vi "DataTranslation_server.vi"(0 "Board type":T1=enum."DT LV-link", 1 "interval scanning":bool, 2 "Client Time":dbl=3399992102.447224, 5 "No of samples+extra":i32=200 min=0 step=1, 7 "Trigger mode":T2, 9 "output polarity":u16(ring)=1 items=["do not change", "positive", "negative"], 11 "Ch & spans":T3[](array[typedef])=[{"high limit (10V)"=10.0, "low limit (-10V)"=-10.0, "Ch No"=0, "Var name"="RV (Vin)", "Use Latest Calib"=FALSE}] {"low limit (-10V)" format="%.3f"; "high limit (10V)" format="%.3f"}, 12 "Actual Sampling rate (Hz)":dbl=10000.0 format="%.2f", 13 "Local Client?":bool=TRUE, 14 "Current Block No":i32) -> (4 "I16 data":i16[][](array[numeric]), 6 "Block Timings":T4={"Started"=3399991568.753699, "Ended"=3399991587.0837474, "Analogue Frequency Hz"=50000.0} {"Analogue Frequency Hz" format="%.2f"}, 10 "group channel settings":T5(array[cluster])=[{"channel"="", "upper input limits"=0.0, "lower input limits"=0.0, "range"=0.0, "polarity"=0, "gain"=0.0, "coupling"=0, "input mode"=0, "scale multiplier"=1.6666666666666668e-07, "scale offset"=0.0}] {"scale offset" format="%#_16f"; "scale multiplier" format="%#_16f"; "input mode" format="%#_16f"; "coupling" format="%#_16f"; "gain" format="%#_16f"; "polarity" format="%#_16f"; "range" format="%#_16f"; "lower input limits" format="%#_16f"; "upper input limits" format="%#_16f"}, 15 "error out":errorcluster={"status"=TRUE, "code"=1172, "source"="Error calling method LvLink2.LvTask.ReadDblData2DAs1D, (System.Reflection.TargetInvocationException: Exception has been thrown by the target of an invocation.\n\tInner Exception: LvLink2.LvException: Timeout) <append><b>LvLink2.LvException</b> in OLReadMultiple2D.vi->DataTranslation_server.vi->Acquire_Data.vi->Get_data.vi->Measurement.vi"})   [LabVIEW 2010]
uses:
  Controls/Block_start_and_end.ctl
  Data_Translation/DataTranslation_global.vi
  Globals/Meas_global.vi
  <userlib>/LV-Link3/PolySubVIs/DtCreateAinChan.vi
  PWA/PWAtasksGLOBAL.vi
  <userlib>/LV-Link3/PolySubVIs/DtOLTimingSetInput.vi
  <userlib>/LV-Link3/PolySubVIs/DtOLReadMultiple2D.vi
  <userlib>/LV-Link3/PolySubVIs/DtOLTriggerDigital.vi
  Controls/Ch_and_Spans.ctl
  Controls/Trigger_Mode.ctl
  Controls/Board_Types.ctl
panel:
  in  "error in":errorcluster
  out "AFG error out":errorcluster
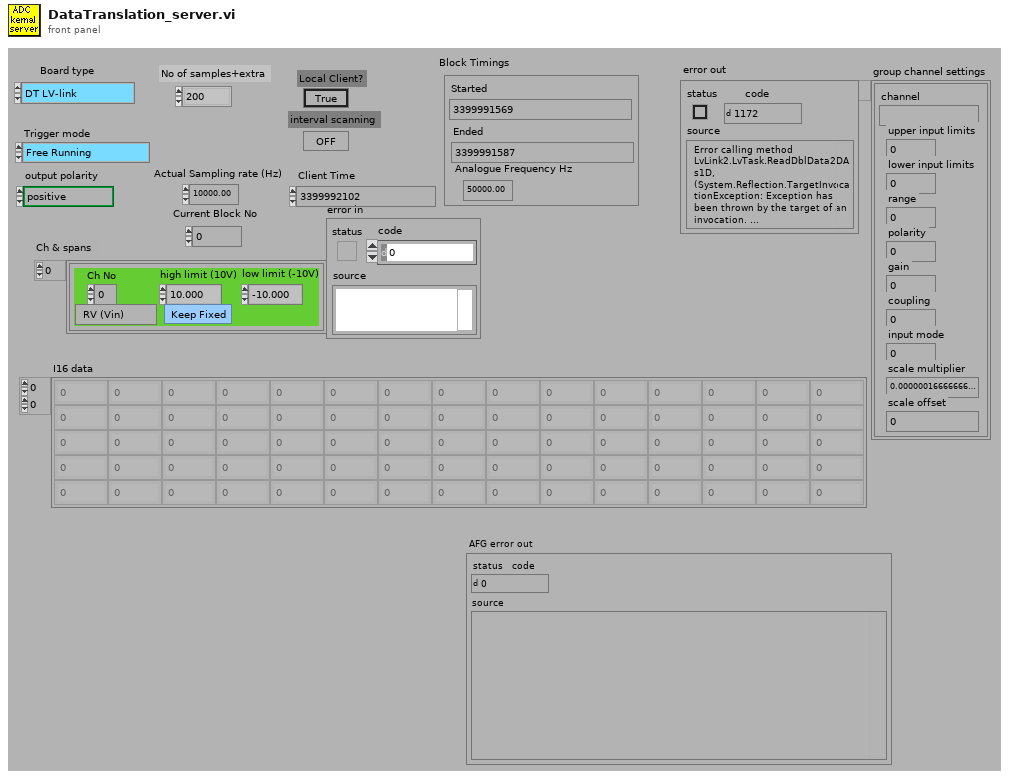
[diagram p1: front panel]
types:
  T1 = typedef "Board_Types.ctl" = enum16{"Simulate", "Local ADAM", "Server ADAM", "NI-DAQmx", "NI-DAQmxBase", "ADC488", "DT LV-link"}
  T2 = typedef "Trigger_Mode.ctl" = enum16{"Free Running", "Start on Trigger", "Trigger Every Block", "Trigger Every Sample"}
  T3 = typedef "Ch_and_Spans.ctl" = cluster{"high limit (10V)":sgl, "low limit (-10V)":sgl, "Ch No":i16, "Var name":string, "Use Latest Calib":bool}
  T4 = typedef "Block_start_and_end.ctl" = cluster{"Started":dbl, "Ended":dbl, "Analogue Frequency Hz":dbl}
  T5 = cluster{"channel":string, "upper input limits":sgl, "lower input limits":sgl, "range":sgl, "polarity":u16, "gain":sgl, "coupling":u16, "input mode":u16, "scale multiplier":dbl, "scale offset":dbl}[]
  T6 = cluster{"channel":string, "upper input limits":sgl, "lower input limits":sgl, "range":sgl, "polarity":u16, "gain":sgl, "coupling":u16, "input mode":u16, "scale multiplier":dbl, "scale offset":dbl}
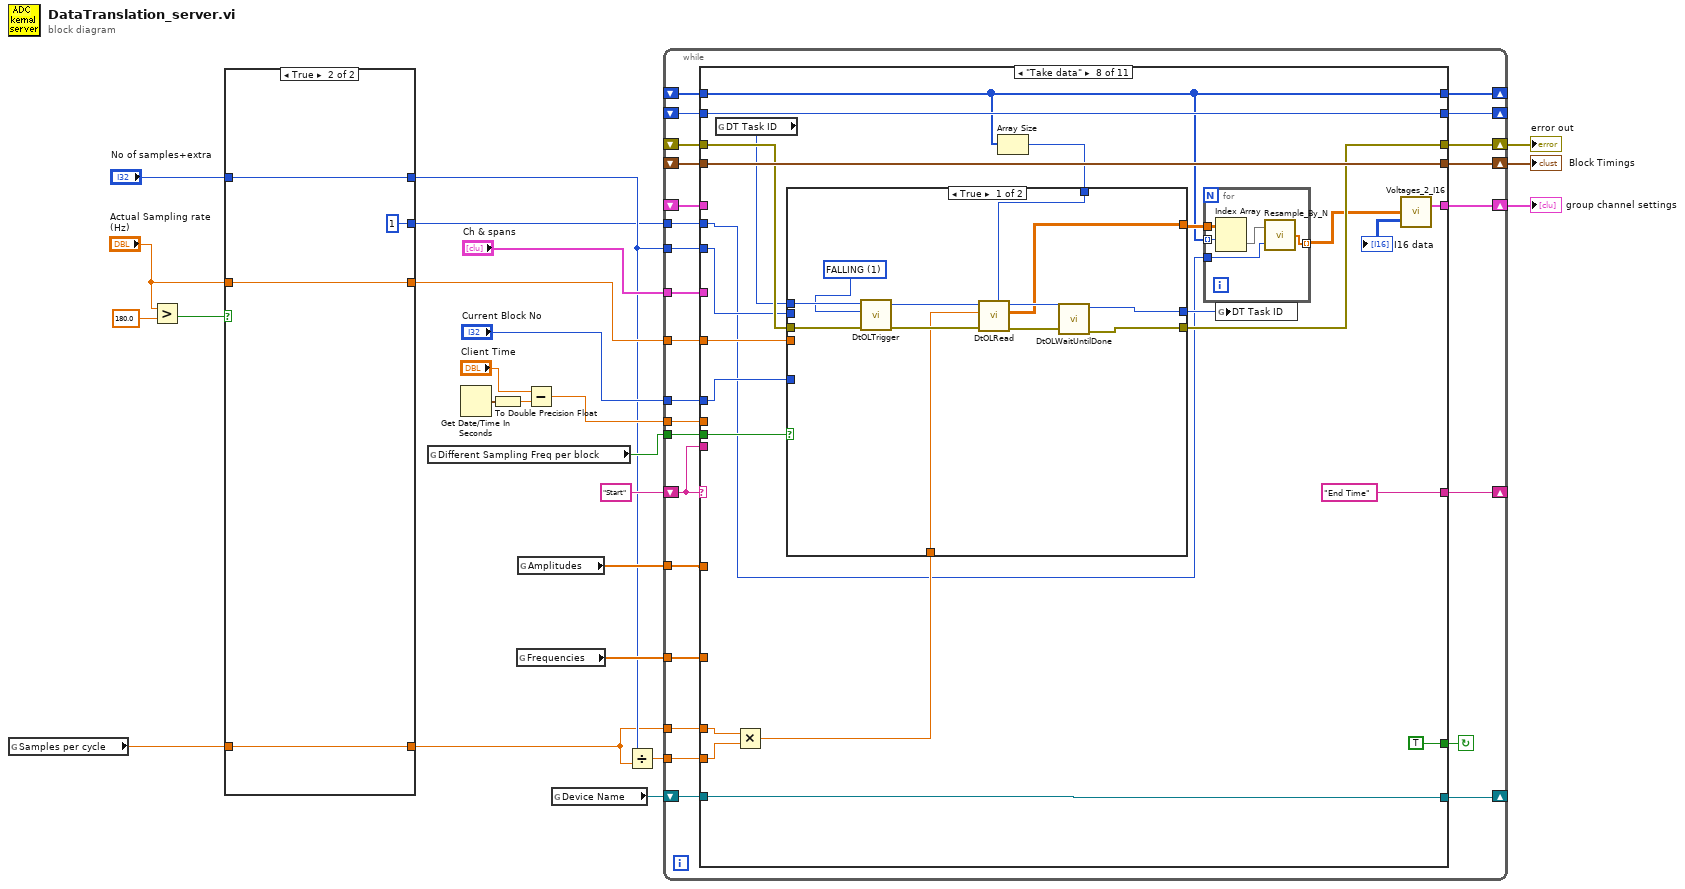
[diagram p0: block diagram]
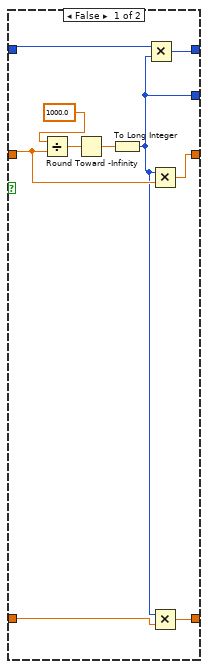
[diagram p2: hidden frame]
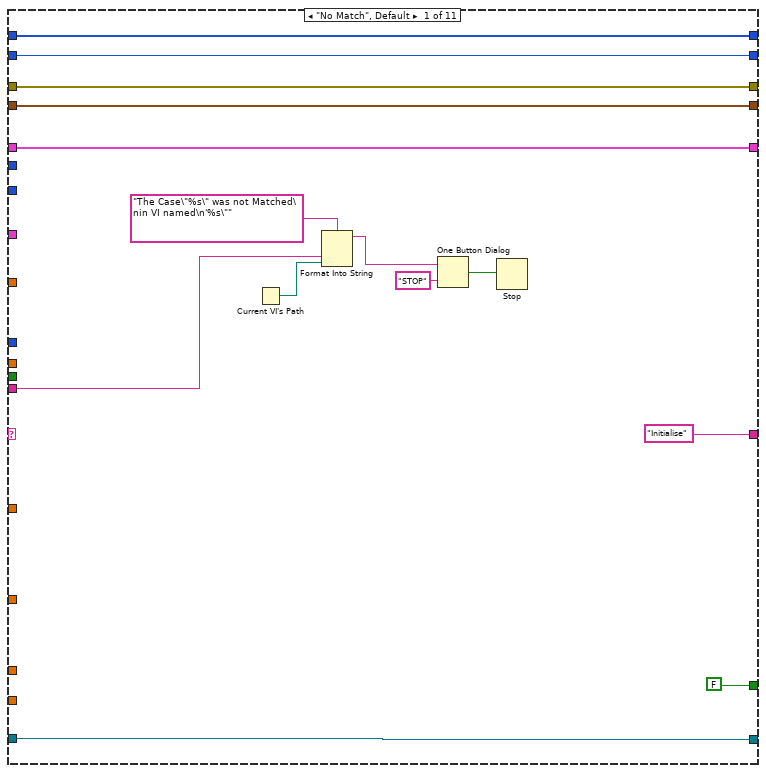
[diagram p3: hidden frame]
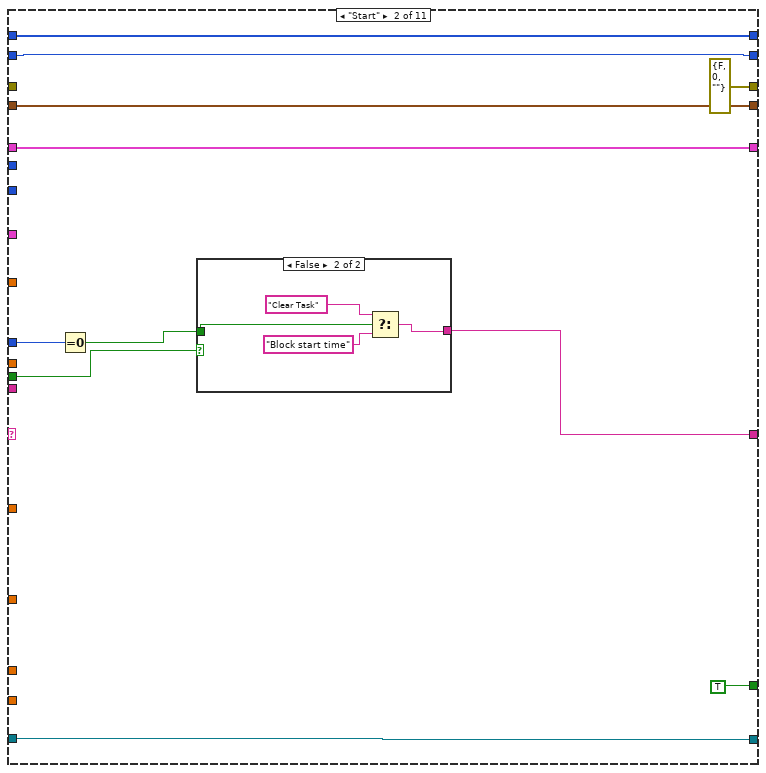
[diagram p4: hidden frame]
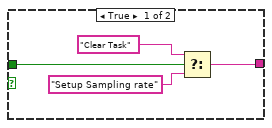
[diagram p5: hidden frame]
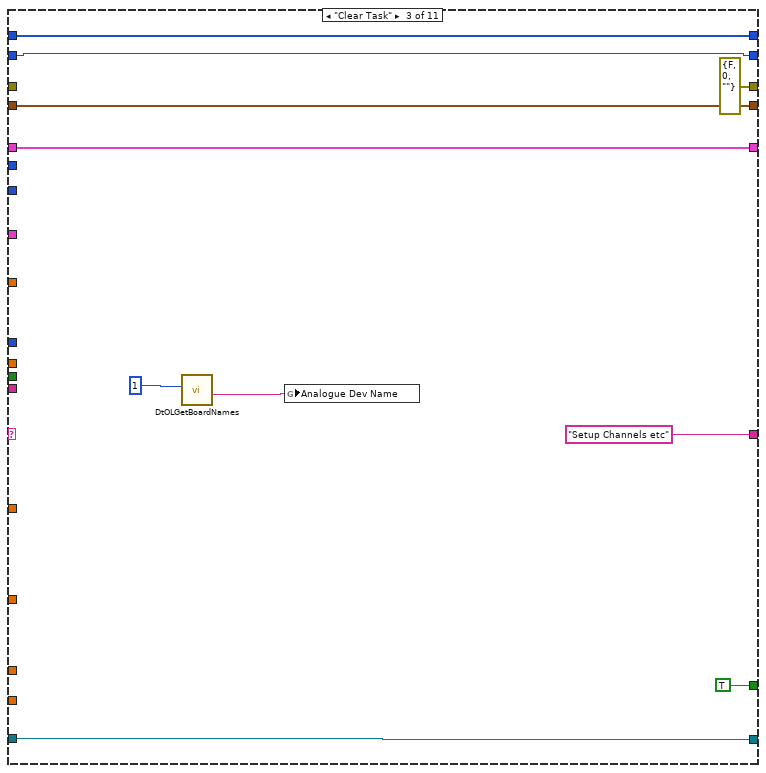
[diagram p6: hidden frame]
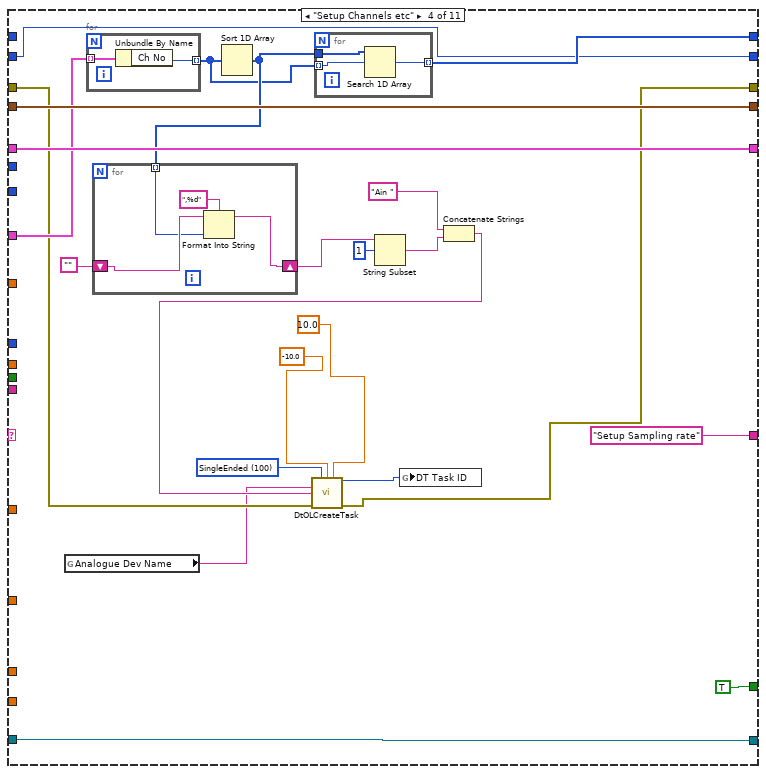
[diagram p7: hidden frame]
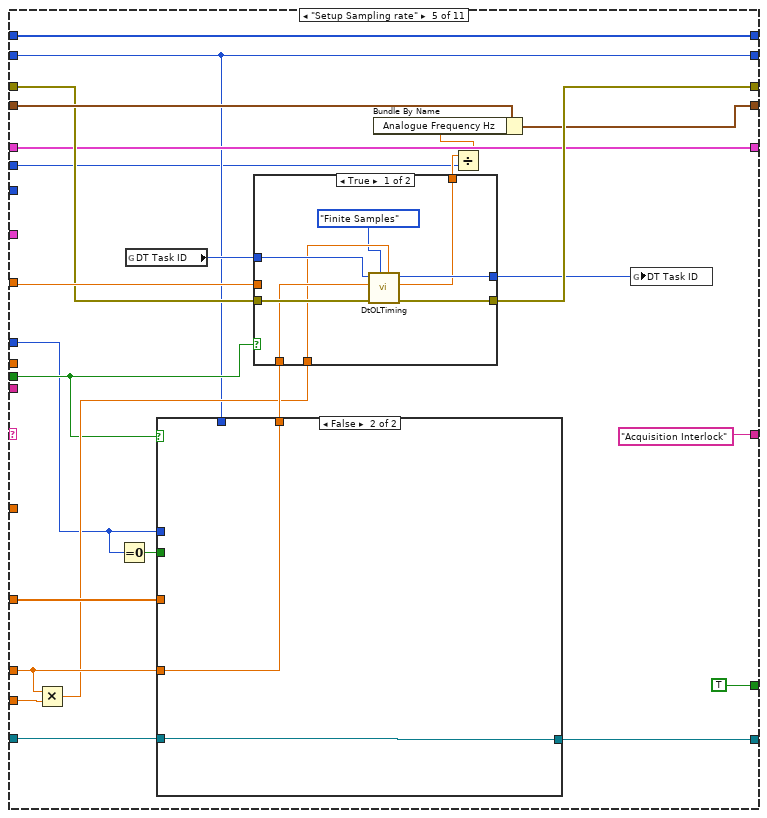
[diagram p8: hidden frame]
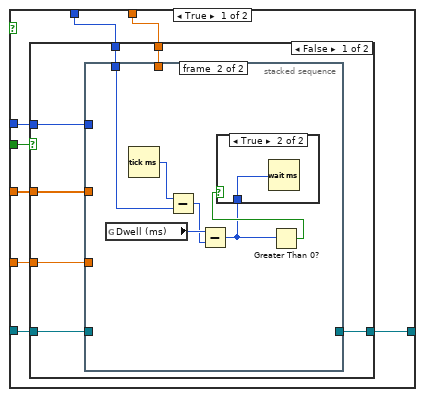
[diagram p9: hidden frame]
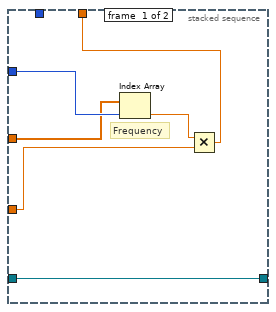
[diagram p10: hidden frame]
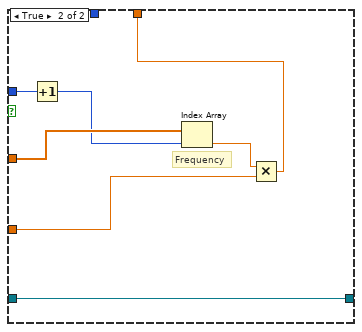
[diagram p12: hidden frame]
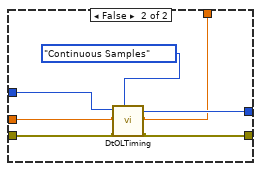
[diagram p13: hidden frame]
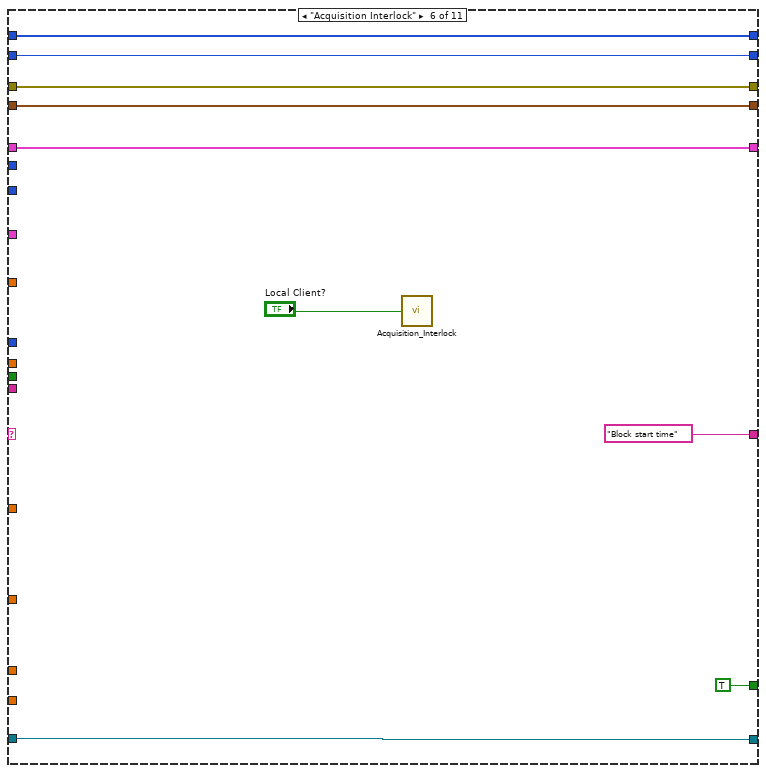
[diagram p14: hidden frame]
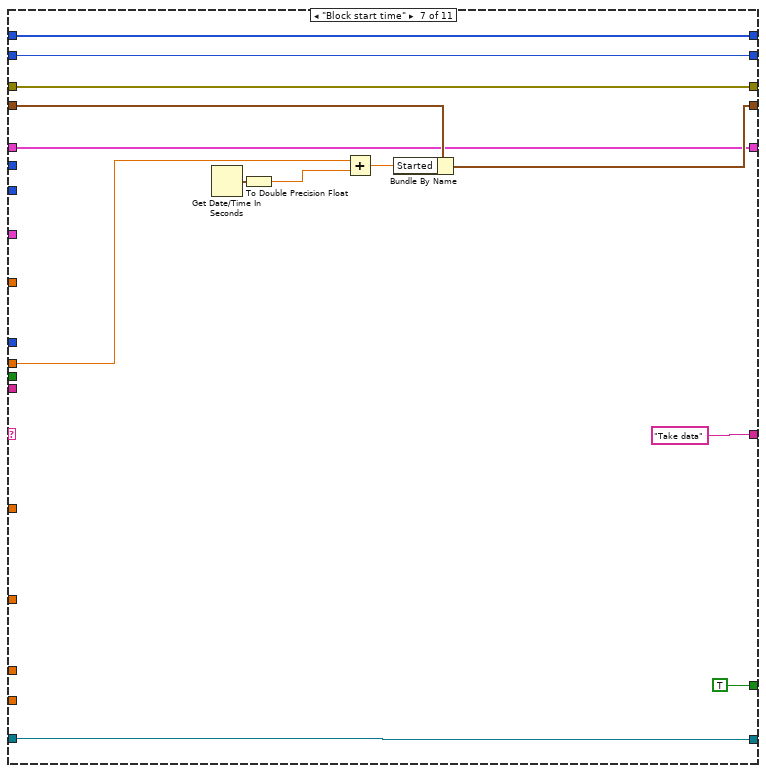
[diagram p15: hidden frame]
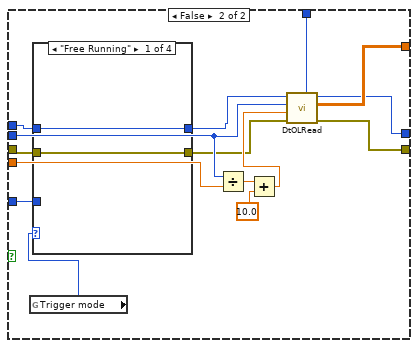
[diagram p16: hidden frame]
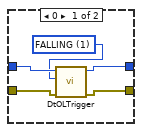
[diagram p18: hidden frame]
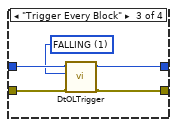
[diagram p19: hidden frame]
diagram:
  n1 = global read "DataTranslation_global.vi" "Samples per cycle"() -> (w2:dbl)
  n2 = Greater?(x="Actual Sampling rate (Hz)", y=180.0) -> (0:w8:bool)
  n3 = case shown="True" w8 {
    tunnel: "Actual Sampling rate (Hz)" -> [w28 w38]
    tunnel: [w29 w38] -> w6
    tunnel: [w31 w37] -> w5
    tunnel: "No of samples+extra" -> [w30 w37]
    tunnel: [w27 w36] -> w3
    tunnel: w2 -> [w26 w36]
    tunnel: [w25 1] -> w1
    frame False {
      n4 = Divide(x=1000.0, y=w28) -> (x/y=w33:dbl)
      n5 = Round Toward -Infinity(1:w33) -> (0:w32:dbl)
      n6 = To Long Integer(number=w32) -> (32bit integer=w25:i32)
      n7 = Multiply(x=w30, y=w25) -> (x*y=w31:i32)
      n8 = Multiply(x=w25, y=w28) -> (x*y=w29:dbl)
      n9 = Multiply(x=w25, y=w26) -> (x*y=w27:dbl)
    }
    frame True {
    }
  }
  n10 = global read "DataTranslation_global.vi" "Different Sampling Freq per block"() -> (w10:bool)
  n11 = Get Date/Time In Seconds() -> (seconds since 1Jan1904=w23:timestamp)
  n12 = To Double Precision Float(number=w23) -> (double precision float=w22:dbl)
  n13 = global read "DataTranslation_global.vi" "Frequencies"() -> (w11:dbl[])
  n14 = global read "DataTranslation_global.vi" "Amplitudes"() -> (w12:dbl[])
  n15 = Subtract(x="Client Time", y=w22) -> (x-y=w20:dbl)
  n16 = global read "DataTranslation_global.vi" "Device Name"() -> (w13:refnum<visa-resource-name>)
  n17 = Divide(x=w5, y=w3) -> (x/y=w15:dbl)
  n18 = while {
    shift-left: "Start" -> [w62]
    shift-right: [w63] -> _
    shift-right: [w53] -> w17
    shift-left: _ -> [w61]
    shift-right: [w52] -> w18
    shift-left: _ -> [w60]
    tunnel: w20 -> [w59]
    tunnel: w6 -> [w58]
    tunnel: w5 -> [w57]
    tunnel: "Current Block No" -> [w56]
    tunnel: "Ch & spans" -> [w55]
    shift-right: [w51] -> w16
    shift-left: _ -> [w54]
    shift-right: [w50] -> _
    shift-left: _ -> [w49]
    tunnel: w3 -> [w47]
    shift-right: [w46] -> _
    shift-left: w13 -> [w48]
    tunnel: w15 -> [w45]
    tunnel: w10 -> [w44]
    tunnel: w12 -> [w43]
    tunnel: w11 -> [w42]
    shift-right: [w41] -> _
    shift-left: _ -> [w40]
    tunnel: w1 -> [w39]
    stop <- w64 continue-if-true
    n19 = case shown="\"Take data\"" w62 {
      tunnel: [FALSE TRUE TRUE TRUE TRUE TRUE TRUE TRUE w318 FALSE FALSE] -> w64
      tunnel: ["Initialise" w85 "Setup Channels etc" "Setup Sampling rate" "Acquisition Interlock" "Block start time" "Take data" "End Time" "Add info to block header" ("f") "End" ("f") "End" ("f")] -> w63
      tunnel: w62 -> [w73 _ _ _ _ _ _ _ _ _ _]
      tunnel: [w70 errorcluster {"status"=FALSE, "code"=0, "source"=""} ("error out") errorcluster {"status"=FALSE, "code"=0, "source"=""} ("error out") w110 w163 w223 w232 w255 w320 w345 w394] -> w53
      tunnel: w61 -> [w70 _ _ w111 w159 w223 w232 w256 w320 w345 w394]
      tunnel: [w68 w88 w106 w122 w160 w221 w236 w257 w325 w343 T4 {"Started"=0.0, "Ended"=0.0, "Analogue Frequency Hz"=1000.0} ("Block Timings")] -> w52
      tunnel: w60 -> [w68 w88 w106 w122 w161 w221 w237 w257 w326 w343 _]
      tunnel: w59 -> [_ _ _ _ _ _ w234 _ w317 _ _]
      tunnel: w58 -> [_ _ _ _ w162 _ _ w249 _ _ _]
      tunnel: w57 -> [_ _ _ _ _ _ _ w250 _ _ _]
      tunnel: w56 -> [_ w87 _ _ w144 _ _ w242 _ w330 _]
      tunnel: w55 -> [_ _ _ w121 _ _ _ _ _ _ _]
      tunnel: [w69 w84 w104 w128 w147 w220 w230 w258 w321 w341 w393] -> w51
      tunnel: w54 -> [w69 w84 w104 w128 w147 w220 w230 _ w321 w342 w393]
      tunnel: [w67 w82 w103 w118 w156 w219 w228 w241 w319 w344 w391] -> w50
      tunnel: w49 -> [w67 w82 w103 _ w156 w219 w228 w241 w319 w344 w391]
      tunnel: w48 -> [w66 w81 w102 w117 w153 w218 w227 w248 w316 w340 w390]
      tunnel: w43 -> [_ _ _ _ _ _ _ _ _ w335 _]
      tunnel: w42 -> [_ _ _ _ w155 _ _ _ _ w336 _]
      tunnel: w47 -> [_ _ _ _ w149 _ _ w246 _ _ _]
      tunnel: [w66 w81 w102 w117 w152 w218 w227 w248 w316 w339 w390] -> w46
      tunnel: w45 -> [_ _ _ _ w150 _ _ w247 _ _ _]
      tunnel: w44 -> [_ w80 _ _ w146 _ _ w244 w318 _ _]
      tunnel: [w65 w79 w101 w116 w145 w217 w226 w243 w315 w332 w389] -> w41
      tunnel: w40 -> [w65 w79 w101 w116 w145 w217 w226 w243 w315 _ w389]
      tunnel: w39 -> [_ _ _ _ w141 _ _ w239 _ _ _]
      frame "No Match", Default {
        n20 = Current VI's Path() -> (path=w72:path)
        n21 = Format Into String(format string="The Case\"%s\" was not Matched\nin VI named\n'%s\"" ("Format String"), w73, w72) -> (resulting string=w76:string)  [unwired: 2 in, 1 out]
        n22 = One Button Dialog(message=w76, button name ("OK")="STOP") -> (true=w74:bool)
        n23 = Stop(stop? (T)=w74) -> ()
      }
      frame "Start" {
        n24 = Equal To 0?(x=w87) -> (x = 0?=w86:bool)
        n25 = case shown="False" w80 {
          tunnel: w86 -> [w91 w95]
          tunnel: [w90 w94] -> w85
          frame True {
            n26 = Select(t="Clear Task", s=w91, f="Setup Sampling rate") -> (s? t:f=w90:string)
          }
          frame False {
            n27 = Select(t="Clear Task", s=w95, f="Block start time") -> (s? t:f=w94:string)
          }
        }
      }
      frame "Clear Task" {
        n28 = call <userlib>:"DtOLGetBoardNames.vi"("Select Board"=u32 1) -> ("Board Name"=w99:string)  [unwired: 8 in, 2 out]
        n29 = global write "PWAtasksGLOBAL.vi" "Analogue Dev Name"(w99) -> ()
      }
      frame "Setup Channels etc" {
        w112 = 100 items=["SingleEnded"=100, "Differential"=101] ("Channel Type")
        n30 = global read "PWAtasksGLOBAL.vi" "Analogue Dev Name"() -> (w108:string)
        n31 = for {
          tunnel: w121 -> [w135] mode=indexing
          tunnel: [w134] -> w119 mode=indexing
          n32 = Unbundle By Name(w135) -> ("Ch No"=w134:i16)
        }
        n33 = Sort 1D Array(array=w119) -> (sorted array=w120:i16[])
        n34 = for {
          shift-right: [w137] -> w127
          shift-left: "" -> [w138]
          tunnel: w120 -> [w136] mode=indexing
          n35 = Format Into String(format string=",%d", initial string=w138, w136) -> (resulting string=w137:string)  [unwired: 1 in, 1 out]
        }
        n36 = for {
          tunnel: w120 -> [w133]
          tunnel: w119 -> [w132] mode=indexing
          tunnel: [w131] -> w118 mode=indexing
          n37 = Search 1D Array(1D array=w133, element=w132) -> (index of element=w131:i32)  [unwired: 1 in]
        }
        n38 = String Subset(string=w127, offset (0)=1) -> (substring=w124:string)  [unwired: 1 in]
        n39 = Concatenate Strings("Ain ", w124) -> (w115:string)
        n40 = call-poly <userlib>:"DtOLCreateTask.vi"("Channel Type"=w112, "Range Min"=-10.0, "Range Max"=10.0, "Board Name"=w108, "Channel"=w115, "error in (no error)"=w111) -> ("Task out"=w109:i32, "error out"=w110:errorcluster)  [unwired: 7 in, 1 out]
        n41 = global write "DataTranslation_global.vi" "DT Task ID"(w109) -> ()
      }
      frame "Setup Sampling rate" {
        n42 = Multiply(x=w149, y=w150) -> (x*y=w148:dbl)
        n43 = Equal To 0?(x=w144) -> (x = 0?=w143:bool)
        n44 = global read "DataTranslation_global.vi" "DT Task ID"() -> (w157:i32)
        n45 = case shown="False" w146 {
          tunnel: w155 -> [w168 _]
          tunnel: [w172 w200] -> w154
          tunnel: w149 -> [w171 w200]
          tunnel: w144 -> [w170 _]
          tunnel: w153 -> [w169 w201]
          tunnel: [w167 w201] -> w152
          tunnel: w145 -> [w166 _]
          tunnel: w143 -> [w165 _]
          frame True {
            n46 = case shown="False" w165 {
              tunnel: [w179 w196] -> w172
              tunnel: w171 -> [w178 w195]
              tunnel: w170 -> [w173 w197]
              tunnel: w169 -> [w177 w194]
              tunnel: w168 -> [w176 w198]
              tunnel: [w175 w194] -> w167
              tunnel: w166 -> [w174 _]
              frame False {
                n47 = stacked-sequence {
                  tunnel: [w185 _] -> w179
                  tunnel: w178 -> [w184 _]
                  tunnel: w173 -> [w183 _]
                  tunnel: w177 -> [w180 _]
                  tunnel: w176 -> [w182 _]
                  tunnel: [w180 _] -> w175
                  tunnel: w174 -> [_ w190]
                  frame #0 {
                    # "Frequency"
                    n48 = Index Array(array=w182, index=w183) -> (element=w181:dbl)
                    n49 = Multiply(x=w181, y=w184) -> (x*y=w185:dbl)
                  }
                  frame #1 {
                    n50 = global read "DataTranslation_global.vi" "Dwell (ms)"() -> (w189:u32)
                    n51 = Tick Count (ms)() -> (millisecond timer value=w191:u32)
                    n52 = Subtract(x=w191, y=w190) -> (x-y=w188:u32)
                    n53 = Subtract(x=w189, y=w188) -> (x-y=w186:u32)
                    n54 = Greater Than 0?(x=w186) -> (x > 0?=w187:bool)
                    n55 = case shown="True" w187 {
                      tunnel: w186 -> [_ w192]
                      frame False {
                      }
                      frame True {
                        n56 = Wait (ms)(milliseconds to wait=w192) -> ()  [unwired: 1 out]
                      }
                    }
                  }
                }
              }
              frame True {
                # "Frequency"
                n57 = Increment(x=w197) -> (x+1=w193:i32)
                n58 = Index Array(array=w198, index=w193) -> (element=w199:dbl)
                n59 = Multiply(x=w199, y=w195) -> (x*y=w196:dbl)
              }
            }
          }
          frame False {
          }
        }
        n60 = case shown="True" w146 {
          tunnel: [w206 w211] -> w163
          tunnel: w162 -> [_ w214]
          tunnel: [w205 w213] -> w142
          tunnel: w159 -> [w207 w212]
          tunnel: [w208 w216] -> w158
          tunnel: w157 -> [w209 w215]
          tunnel: w154 -> [w204 _]
          tunnel: w148 -> [w203 _]
          frame True {
            n61 = call-poly <userlib>:"DtOLTiming.vi"("Samples Per Channel"=w203, "Sample Mode"=enum16{"Finite Samples", "Continuous Samples"}."Finite Samples", "error in (no error)"=w207, "Sample Freq (Hz)"=w204, "Task in"=w209) -> ("error out"=w206:errorcluster, "Actual Sample Freq"=w205:dbl, "Task out"=w208:i32)  [unwired: 3 in, 1 out]
          }
          frame False {
            n62 = call-poly <userlib>:"DtOLTiming.vi"("Sample Mode"=enum16{"Finite Samples", "Continuous Samples"}."Continuous Samples", "error in (no error)"=w212, "Sample Freq (Hz)"=w214, "Task in"=w215) -> ("error out"=w211:errorcluster, "Actual Sample Freq"=w213:dbl, "Task out"=w216:i32)  [unwired: 4 in, 1 out]
          }
        }
        n63 = Divide(x=w142, y=w141) -> (x/y=w140:dbl)
        n64 = Bundle By Name(cluster=w161, "Analogue Frequency Hz"=w140) -> (w160:T4)
        n65 = global write "DataTranslation_global.vi" "DT Task ID"(w158) -> ()
      }
      frame "Acquisition Interlock" {
        n66 = call "Acquisition_Interlock.vi"("Local Control"="Local Client?") -> ()
      }
      frame "Block start time" {
        n67 = Get Date/Time In Seconds() -> (seconds since 1Jan1904=w238:timestamp)
        n68 = To Double Precision Float(number=w238) -> (double precision float=w235:dbl)
        n69 = Add(x=w234, y=w235) -> (x+y=w233:dbl)
        n70 = Bundle By Name(cluster=w237, "Started"=w233) -> (w236:T4)
      }
      frame "Take data" {
        n71 = global read "DataTranslation_global.vi" "DT Task ID"() -> (w253:i32)
        n72 = Multiply(x=w246, y=w247) -> (x*y=w245:dbl)
        n73 = Array Size(array=w241) -> (size(s)=w240:i32)
        n74 = case shown="True" w244 {
          tunnel: w256 -> [w273 w283]
          tunnel: [w270 w277] -> w255
          tunnel: [w267 w275] -> w254
          tunnel: w253 -> [w266 w284]
          tunnel: [w264 w276] -> w252
          tunnel: w250 -> [_ w280]
          tunnel: w249 -> [_ w288]
          tunnel: w245 -> [w263 _]
          tunnel: w242 -> [_ w282]
          tunnel: w240 -> [w262 w274]
          frame True {
            w265 = 1 items=["RISING", "FALLING"] ("External Trigger Polarity")
            n75 = call-poly <userlib>:"DtOLTrigger.vi"("error in (no error)"=w273, "External Trigger Polarity"=w265, "Task in"=w266) -> ("error out"=w272:errorcluster, "Task out"=w269:i32)  [unwired: 7 in]
            n76 = call-poly <userlib>:"DtOLRead.vi"("Number Chan to Read"=w262, "error in (no error)"=w272, "Samples Per Channel"=w263, "Task in"=w269) -> ("error out"=w271:errorcluster, "2D Data out"=w264:dbl[][], "Task out"=w268:i32)  [unwired: 3 in, 2 out]
            n77 = call <userlib>:"DtOLWaitUntilDone.vi"("error in"=w271, "Task in"=w268) -> ("error out"=w270:errorcluster, "Task out"=w267:i32)  [unwired: 8 in]
          }
          frame False {
            n78 = global read "Meas_global.vi" "Trigger mode"() -> (w285:T2)
            n79 = case shown="\"Free Running\"" w285 {
              tunnel: [w290 w292 w306 w309] -> w281
              tunnel: w284 -> [w290 w294 w307 w309]
              tunnel: [w289 w291 w303 w308] -> w278
              tunnel: w283 -> [w289 w293 w304 w308]
              tunnel: w282 -> [_ w295 _ _]
              frame "Free Running" {
              }
              frame "Start on Trigger" {
                n80 = case shown="1, Default" w295 {
                  tunnel: w294 -> [w300 w302]
                  tunnel: w293 -> [w298 w301]
                  tunnel: [w296 w302] -> w292
                  tunnel: [w297 w301] -> w291
                  frame 0 {
                    w299 = 1 items=["RISING", "FALLING"] ("External Trigger Polarity")
                    n81 = call-poly <userlib>:"DtOLTrigger.vi"("error in (no error)"=w298, "External Trigger Polarity"=w299, "Task in"=w300) -> ("error out"=w297:errorcluster, "Task out"=w296:i32)  [unwired: 7 in]
                  }
                  frame 1, Default {
                  }
                }
              }
              frame "Trigger Every Block" {
                w305 = 1 items=["RISING", "FALLING"] ("External Trigger Polarity")
                n82 = call-poly <userlib>:"DtOLTrigger.vi"("error in (no error)"=w304, "External Trigger Polarity"=w305, "Task in"=w307) -> ("error out"=w303:errorcluster, "Task out"=w306:i32)  [unwired: 7 in]
              }
              frame "Trigger Every Sample" {
              }
            }
            n83 = Divide(x=w280, y=w288) -> (x/y=w286:dbl)
            n84 = Add(x=w286, y=10.0) -> (x+y=w279:dbl)
            n85 = call-poly <userlib>:"DtOLRead.vi"("Number Chan to Read"=w274, "error in (no error)"=w278, "Timeout"=w279, "Samples Per Channel"=w280, "Task in"=w281) -> ("error out"=w277:errorcluster, "2D Data out"=w276:dbl[][], "Task out"=w275:i32)  [unwired: 2 in, 2 out]
          }
        }
        n86 = for {
          tunnel: w241 -> [w314] mode=indexing
          tunnel: w252 -> [w313]
          tunnel: [w311] -> w251 mode=indexing
          tunnel: w239 -> [w310]
          n87 = Index Array(array=w313, index (row)=w314) -> (element=w312:dbl[])  [unwired: 1 in]
          n88 = call "Resample_By_N.vi"("Resample Factor"=w310, "Array In"=w312) -> ("Array Out"=w311:dbl[])
        }
        n89 = global write "DataTranslation_global.vi" "DT Task ID"(w254) -> ()
        n90 = call "Voltages_2_I16.vi"("Voltages"=w251) -> ("Group Channel Settings"=w258:T5, "I16 data"=→"I16 data":i16[][])
      }
      frame "End Time" {
        # "Final transpose to get 2D data output correctly"
        n91 = Get Date/Time In Seconds() -> (seconds since 1Jan1904=w327:timestamp)
        n92 = To Double Precision Float(number=w327) -> (double precision float=w324:dbl)
        n93 = Add(x=w317, y=w324) -> (x+y=w323:dbl)
        n94 = Bundle By Name(cluster=w326, "Ended"=w323) -> (w325:T4)
      }
      frame "Add info to block header" {
        n95 = global read "Meas_global.vi" "Requested No of blocks"() -> (w333:i32)
        n96 = Index Array(array=w335, index=w330) -> (element=w338:dbl)
        n97 = Index Array(array=w336, index=w330) -> (element=w337:dbl)
        n98 = Decrement(x=w333) -> (x-1=w331:i32)
        n99 = for {
          tunnel: w342 -> [w376] mode=indexing
          tunnel: [w375] -> w341 mode=indexing
          tunnel: w338 -> [w374]
          tunnel: w337 -> [w373]
          i -> [w377]
          n100 = case shown="0" w377 {
            tunnel: w376 -> [w387 w388]
            tunnel: [w381 w388] -> w375
            tunnel: w374 -> [w384 _]
            tunnel: w373 -> [w383 _]
            frame 0 {
              n101 = call "Value_to_string.vi"("Value"=w384, "Label for value"="Function_Generator_Amplitude") -> ("Output string"=w380:string)  [unwired: 1 in]
              n102 = call "Value_to_string.vi"("precision"="0", "Value"=w383, "Label for value"="Function_Generator_Frequency") -> ("Output string"=w379:string)
              n103 = Concatenate Strings(w380, w379) -> (w378:string)
              n104 = Bundle By Name(cluster=w387, "channel"=w378) -> (w381:T6)
            }
            frame 1, Default {
            }
          }
        }
        n105 = Equal?(x=w330, y=w331) -> (x = y?=w334:bool)
        n106 = case shown="False" w334 {
          tunnel: w340 -> [w360 w370]
          tunnel: [w351 w368] -> w339
          tunnel: [w353 w369] -> w328
          tunnel: w336 -> [w356 w371]
          tunnel: w335 -> [w357 w372]
          tunnel: w330 -> [w355 _]
          tunnel: [w357 w372] -> _
          tunnel: [w356 w371] -> _
          tunnel: "error in" -> [w348 w366]
          frame False {
            w361 = "SOUR1" ("input 1")
            w364 = ":%s:FREQ %.;%g;"  # Frequency Command
            w365 = ":%s:VOLT %.;%g;"  # Amplitude Command
            n107 = Increment(x=w355) -> (x+1=w354:i32)
            n108 = Index Array(array=w357, index=w354) -> (element=w359:dbl)
            n109 = Index Array(array=w356, index=w354) -> (element=w358:dbl)
            n110 = Format Into String(format string=w364, w361, w358) -> (resulting string=w362:string)  [unwired: 2 in, 1 out]
            n111 = Format Into String(format string=w365, initial string=w362, w361, w359) -> (resulting string=w363:string)  [unwired: 1 in, 1 out]
            n112 = VISA Write(VISA resource name=w360, write buffer=w363, error in (no error)=w348) -> (VISA resource name out=w352:refnum<visa-resource-name>, error out=w350:errorcluster)  [unwired: 1 out]
            n113 = VISA Write(VISA resource name=w352, write buffer="OUTP1:STAT ON", error in (no error)=w350) -> (VISA resource name out=w351:refnum<visa-resource-name>, error out=w353:errorcluster)  [unwired: 1 out]
          }
          frame True {
            n114 = VISA Write(VISA resource name=w370, write buffer="OUTP1:STAT OFF", error in (no error)=w366) -> (VISA resource name out=w368:refnum<visa-resource-name>, error out=w369:errorcluster)  [unwired: 1 out]
          }
        }
        "AFG error out" <- w328
        n115 = Tick Count (ms)() -> (millisecond timer value=w332:u32)
      }
      frame "Extra case" {
      }
    }
  }
  "Block Timings" <- w18
  "error out" <- w17
  "group channel settings" <- w16
